vi "TagDB-Status.vi"(8 "error in (no error)":errorcluster, 10 "return elements? (F)":bool, 11 "DB Ref":T1) -> (0 "error out":errorcluster, 1 "Item Change Timestamp":timestamp, 2 "Global Change Timestamp":timestamp, 3 "DB Ref(dup)":T1, 4 "DB items":string[](array[string]), 5 "db name":string)   [LabVIEW 2017, in "TagDB(DEV).lvlib"]
doc: "[Covers: REQ_API_Status]"
uses:
  TagDB(DEV).lvlib
  Typedef/TagDB.ctl
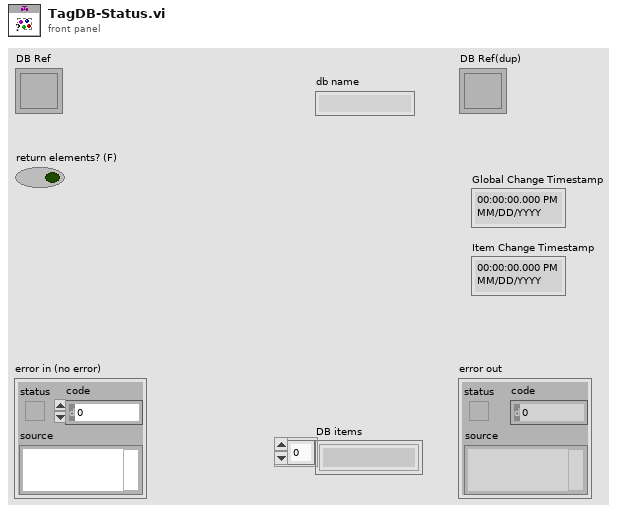
[diagram p1: front panel]
types:
  T1 = typedef "TagDB(DEV).lvlib/TagDB.ctl" = refnum<k1>
  T2 = typedef "TagContainer.lvlib/tagcontainer-data.ctl" = cluster{"tag-map":variant, "timestamp-map":variant, "namecacher-map":variant, "DataTypeCacher-map":variant, "Tag Adding Lock?":bool, "Global Change Timestamp":timestamp, "Item Change Timestamp":timestamp, "name":string}
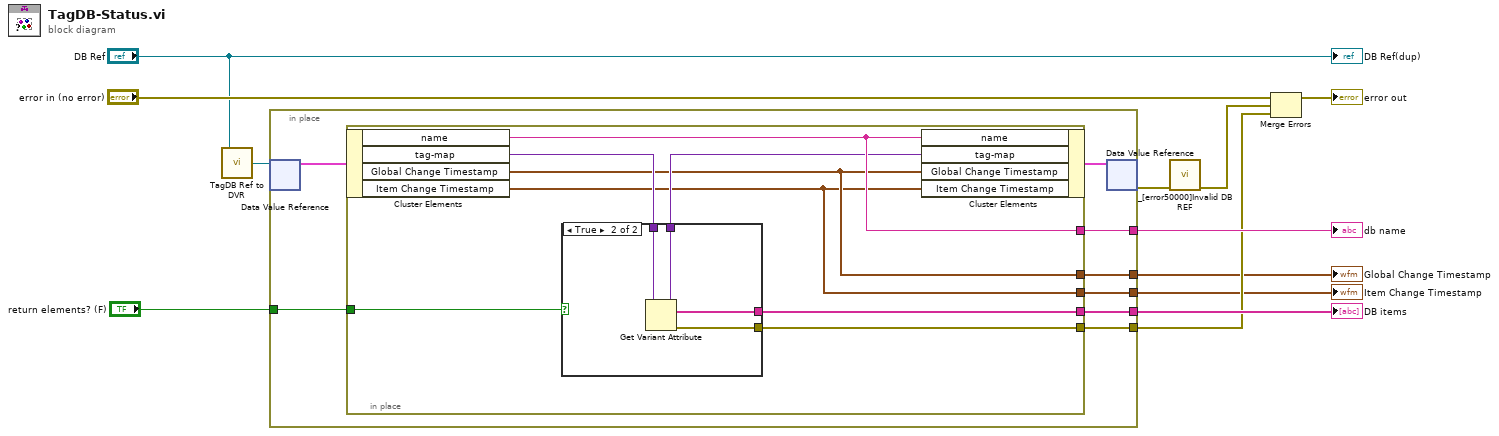
[diagram p0: block diagram]
diagram:
  n1 = call "TagDB Ref to DVR.vi"("TagDB"="DB Ref") -> ("DVR"=w6:refnum<data-value>)  [unwired: 4 in]
  n2 = in-place {
    in-place-border: [w20] -> w8
    in-place-border: [w19] -> w3
    in-place-border: "return elements? (F)" -> [w18]
    in-place-border: [w17] -> w7
    in-place-border: [w15] -> w2
    in-place-border: [w14] -> w1
    n3 = in-place-dvr #1(w6) -> (w16:T2)  [unwired: 1 out]
    n4 = in-place {
      in-place-border: [w28] -> w20
      in-place-border: [w27] -> w19
      in-place-border: w18 -> [w26]
      in-place-border: [w24] -> w17
      in-place-border: [w22] -> w15
      in-place-border: [w21] -> w14
      n5 = in-place-cluster #2(w16) -> ("name"=w24:string, "tag-map"=w25:variant, "Global Change Timestamp"=w22:timestamp, "Item Change Timestamp"=w21:timestamp)
      n6 = case shown="True" w26 {
        tunnel: w25 -> [w29 w33]
        tunnel: [_ w32] -> w28
        tunnel: [_ w31] -> w27
        tunnel: [w29 w30] -> w23
        frame False {
        }
        frame True {
          n7 = Get Variant Attribute(Variant=w33) -> (duplicate Variant=w30:variant, names=w32:string[], error out=w31:errorcluster)  [unwired: 3 in, 1 out]
        }
      }
      n8 = in-place-cluster #2("name"=w24, "tag-map"=w23, "Global Change Timestamp"=w22, "Item Change Timestamp"=w21) -> (w13:T2)
    }
    n9 = in-place-dvr #1(w13) -> (w5:errorcluster)  [unwired: 1 out]
  }
  "db name" <- w7
  "Global Change Timestamp" <- w2
  "Item Change Timestamp" <- w1
  "DB items" <- w8
  n10 = call "_[error50000]Invalid DB REF.vi"("error in (no error)"=w5) -> ("error out"=w4:errorcluster)  [unwired: 10 in]
  n11 = Merge Errors("error in (no error)", w4, w3) -> (→"error out":errorcluster)
  "DB Ref(dup)" <- "DB Ref"
